vi "saveXML.vi"(8 "error in (no error)":errorcluster, 10 "Path":path, 11 "NativeXML in":refnum<class "NativeXML.lvclass">) -> (0 "error out":errorcluster, 3 "NativeXML out":refnum<class "NativeXML.lvclass">)   [LabVIEW 2011, in "Tools.lvlib" / "xml.lvlib" / "NativeXML.lvclass"]
uses:
  NativeXML.lvclass
  NativeXML.lvclass/NativeXML.ctl
  <vilib>/xml/NI_XML.lvlib
  Program Files/National Instruments/LabVIEW 2011/resource/objmgr/DOMUserDefRef.rc
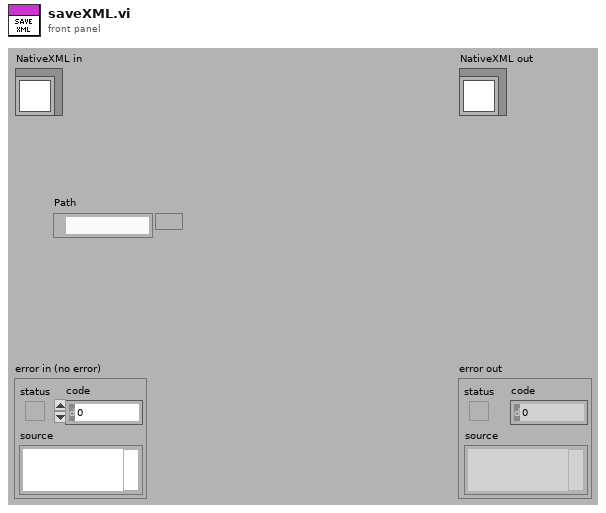
[diagram p1: front panel]
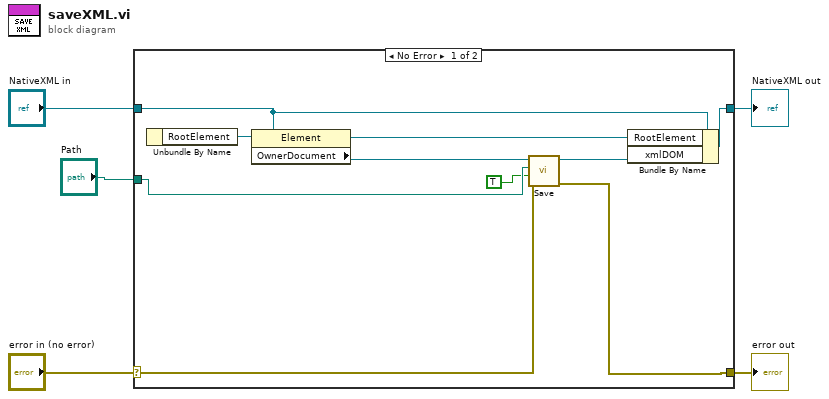
[diagram p0: block diagram]
diagram:
  n1 = case shown="No Error" "error in (no error)" {
    selector: "error in (no error)" -> [w7 w17]
    tunnel: [w9 w17] -> w4
    tunnel: [w10 w16] -> w2
    tunnel: "NativeXML in" -> [w11 w16]
    tunnel: "Path" -> [w15 _]
    frame No Error {
      n2 = Unbundle By Name(w11) -> ("RootElement"=w13:refnum<k20>)
      n3 = property class="Element"(reference=w13) -> (reference out=w12:refnum<k20>, "OwnerDocument"=w6:refnum<k20>)  [unwired: 1 in, 1 out]
      n4 = call <vilib>:"Save.vi"("error in (no error)"=w7, "overwrite file (True)"=TRUE, "XML file path"=w15, "DOM document in"=w6) -> ("error out"=w9:errorcluster, "DOM document out"=w8:refnum<k20>)  [unwired: 5 in, 1 out]
      n5 = Bundle By Name(cluster=w11, "RootElement"=w12, "xmlDOM"=w8) -> (w10:refnum<class "NativeXML.lvclass">)
    }
    frame Error {
    }
  }
  "error out" <- w4
  "NativeXML out" <- w2
